vi "Silvermax_restart.vi"(4 "error in (no error)":errorcluster, 6 "Motor #":u8) -> (0 "error out":errorcluster, 2 "Motor # dup":u8)   [LabVIEW 2015]
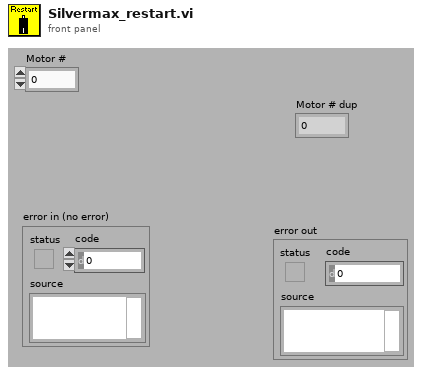
[diagram p1: front panel]
types:
  T1 = enum16{"POL (0)", "CPL (1)", "HLT (2)", "STP (3)", "RST (4)", "RVN (5)", "RPB (6)", "CLP (8)", "SDL (9)", "RUN (10)", "WRI (11)", "RRG (12)", "SPR (13)", "LPR (14)", "VMI (15)", "SSP (17)", "SSE (18)", "RIS (20)", "RIO (21)", "IMW (25)", "END (128)", "MAV (134)", "MRV (135)", "JRE (137)", "WCL (138)", "WCW (139)", "DLY (140)", "WDL (141)", "GCL (142)", "GOP (143)", "ZTG (144)", "ZTP (145)", "TTP (146)", "CME (147)", "CTC (148)", "TQL (149)", "AHC (150)", "ERL (151)", "OLP (152)", "WRP (154)", "IDT (155)", "LRP (156)", "VMP (159)", "RAV (160)", "RRV (161)", "JMP (162)", "JOI (162)", "CIS (163)", "CKS (164)", "CLC (165)", "KMC (167)", "MCT (168)", "FLC (169)", "EEM (170)", "DDB (171)", "DEM (171)", "PAC (172)", "ADL (173)", "BRT (174)", "MAT (176)", "MRT (177)", "RAT (178)", "RRT (179)", "SSD (180)", "KMR (181)", "KED (182)", "KDD (183)", "DIR (184)", "PRO (185)", "SIF (186)", "EDL (187)", "CIO (188)", "MDS (189)", "MDC (190)", "MDT (191)", "SEE (192)", "ARI (193)", "WBS (194)", "SCF (195)", "RSM (196)", "RLM (197)", "RSN (198)", "RLN (199)", "PCL (201)", "PCI (201)", "PRT (202)", "PRI (202)", "WBE (204)", "SOB (205)", "COB (206)", "ACR (207)", "PLR (208)", "CAI (211)", "LVT (212)", "OVT (213)", "MTT (214)", "CLC (215)", "PIM (216)", "VIM (217)", "TIM (218)", "AHM (219)", "SSL (221)", "TRU (222)", "RSD (223)", "EMT (225)", "DMT (226)", "EMD (227)", "DMD (228)", "HSM (229)", "AHD (230)", "PCM (231)", "PCG (232)", "XRV (233)", "XAV (234)", "XRT (235)", "XAT (236)", "GOC (237)", "JNA (238)", "JOR (239)", "PMC (240)", "PMV (241)", "PMX (242)", "DLC (243)", "SLC (244)", "PCP (245)", "ATR (248)", "PMO (249)", "JAN (250)", "EDH (251)", "DIF (252)", "IMS (253)", "IMQ (254)"}
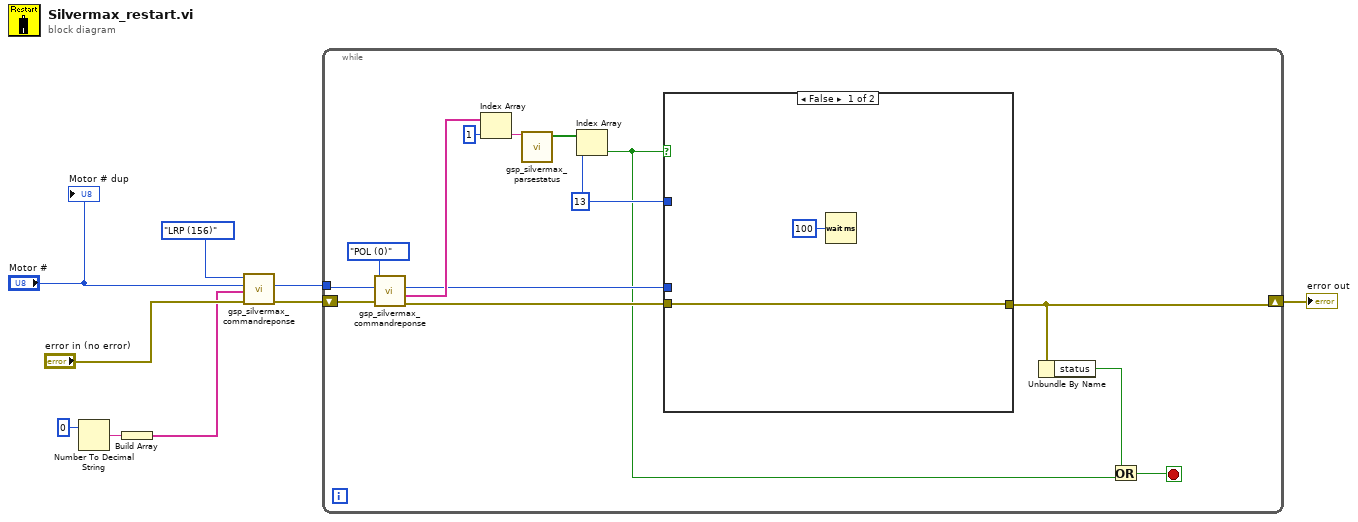
[diagram p0: block diagram]
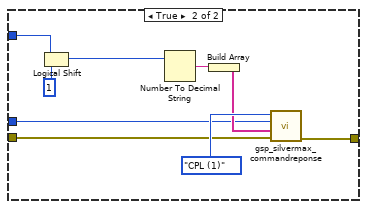
[diagram p2: hidden frame]
diagram:
  n1 = Number To Decimal String(number=0) -> (decimal integer string=w3:string)  [unwired: 1 in]
  n2 = Build Array(w3) -> (w1:string[])
  n3 = call "gsp_silvermax_commandreponse.vi"("error in (no error)"="error in (no error)", "Parameters (none)"=w1, "Motor #"="Motor #", "Command"=T1."LRP (156)") -> ("error out"=w4:errorcluster, "Motor # dup"=w7:u8)  [unwired: 2 out]
  n4 = while {
    tunnel: w7 -> [w20]
    shift-right: [w11] -> w6
    shift-left: w4 -> [w21]
    stop <- w23 stop-if-true
    w13 = 13 ("index")
    n5 = call "gsp_silvermax_commandreponse.vi"("error in (no error)"=w21, "Motor #"=w20, "Command"=T1."POL (0)") -> ("error out"=w15:errorcluster, "Parameter Array"=w19:string[], "Motor # dup"=w14:u8)  [unwired: 1 in, 1 out]
    n6 = Index Array(array=w19, index=1) -> (element=w17:string)
    n7 = call "gsp_silvermax_parsestatus.vi"("Status Word in Hex"=w17) -> ("Boolean Array"=w16:bool[])  [unwired: 6 in]
    n8 = Index Array(array=w16, index=w13) -> (element=w10:bool)
    n9 = case shown="False" w10 {
      tunnel: w15 -> [w25 w29]
      tunnel: w14 -> [_ w28]
      tunnel: w13 -> [_ w27]
      tunnel: [w25 w26] -> w11
      frame False {
        n10 = Wait (ms)(milliseconds to wait=u32 100) -> ()  [unwired: 1 out]
      }
      frame True {
        n11 = Logical Shift(y=w27, x=u16 1) -> (x << y=w30:u16)
        n12 = Number To Decimal String(number=w30) -> (decimal integer string=w33:string)  [unwired: 1 in]
        n13 = Build Array(w33) -> (w31:string[])
        n14 = call "gsp_silvermax_commandreponse.vi"("error in (no error)"=w29, "Parameters (none)"=w31, "Motor #"=w28, "Command"=T1."CPL (1)") -> ("error out"=w26:errorcluster)  [unwired: 3 out]
      }
    }
    n15 = Unbundle By Name(w11) -> ("status"=w12:bool)
    n16 = Or(x=w12, y=w10) -> (x .or. y?=w23:bool)
  }
  "error out" <- w6
  "Motor # dup" <- "Motor #"
